vi "Teleop Fingers.vi"(10 "Joystick Data":T2, 11 "Arm Out":T1) -> ()   [LabVIEW 2013]
uses:
  Joystick Data.ctl
  <vilib>/Rock Robotics/WPI/Solenoid/WPI_SolenoidValue.ctl
  <vilib>/Rock Robotics/WPI/Solenoid/WPI_SolenoidSetEnum.vi
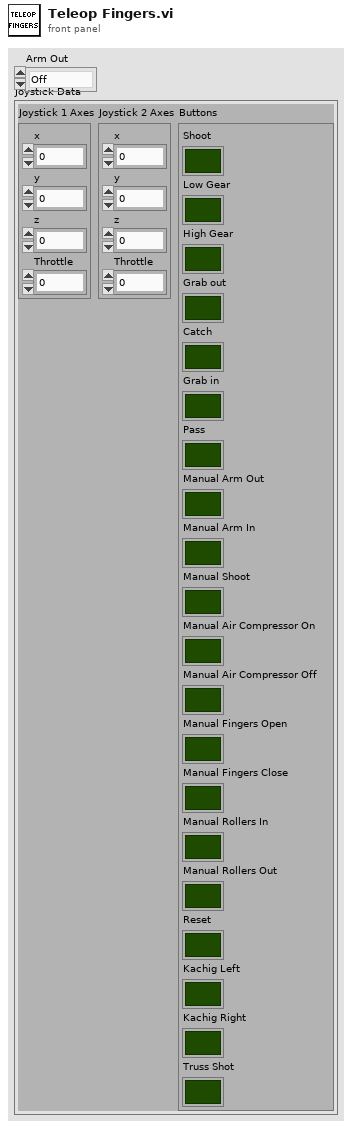
[diagram p1: front panel]
types:
  T1 = typedef "WPI_SolenoidValue.ctl" = enum16{"Off", "On", "Forward", "Reverse"}
  T2 = typedef "Joystick Data.ctl" = cluster{"Joystick 1 Axes":cluster{"x":dbl, "y":dbl, "z":dbl, "Throttle":dbl}, "Joystick 2 Axes":cluster{"x":dbl, "y":dbl, "z":dbl, "Throttle":dbl}, "Buttons":cluster{"Shoot":bool, "Low Gear":bool, "High Gear":bool, "Grab out":bool, "Catch":bool, "Grab in":bool, "Pass":bool, "Manual Arm Out":bool, "Manual Arm In":bool, "Manual Shoot":bool, "Manual Air Compressor On":bool, "Manual Air Compressor Off":bool, "Manual Fingers Open":bool, "Manual Fingers Close":bool, "Manual Rollers In":bool, "Manual Rollers Out":bool, "Reset":bool, "Kachig Left":bool, "Kachig Right":bool, "Truss Shot":bool}}
  T3 = typedef "WPI_SolenoidDevRef.ctl" = cluster{"DevStatus":errorcluster, "Solenoid Module":T4, "Forward Solenoid Channel":T5, "Reverse Solenoid Channel":T5}
  T4 = typedef "FPGA_TypedefSolenoidModule.ctl" = enum16{"Solenoid Module 1", "Solenoid Module 2"}
  T5 = typedef "WPI_SolenoidChannel.ctl" = enum8{"Solenoid 1", "Solenoid 2", "Solenoid 3", "Solenoid 4", "Solenoid 5", "Solenoid 6", "Solenoid 7", "Solenoid 8", "Invalid"}
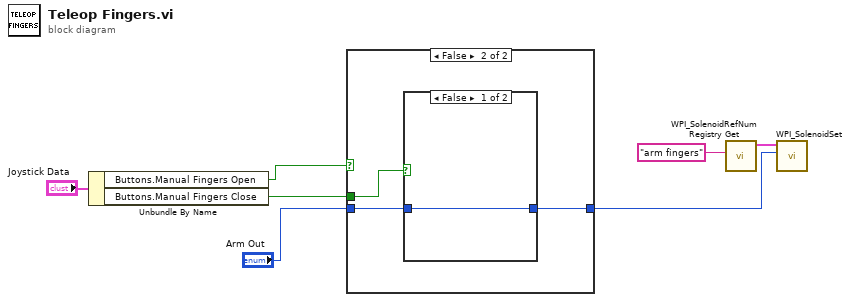
[diagram p0: block diagram]
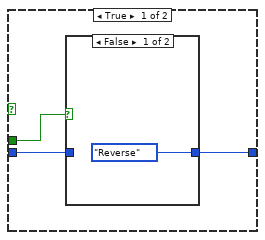
[diagram p2: hidden frame]
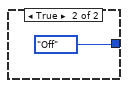
[diagram p3: hidden frame]
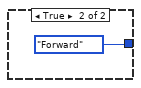
[diagram p4: hidden frame]
diagram:
  n1 = Unbundle By Name("Joystick Data") -> ("Buttons.Manual Fingers Open"=w4:bool, "Buttons.Manual Fingers Close"=w3:bool)
  n2 = case shown="False" w4 {
    tunnel: w3 -> [w10 w15]
    tunnel: "Arm Out" -> [w9 w14]
    tunnel: [w8 w13] -> w1
    frame True {
      n3 = case shown="False" w10 {
        tunnel: [WPI_SolenoidValue."Reverse" ("Arm Out") WPI_SolenoidValue."Off" ("Arm Out")] -> w8
        tunnel: w9 -> [_ _]
        frame False {
        }
        frame True {
        }
      }
    }
    frame False {
      n4 = case shown="False" w15 {
        tunnel: w14 -> [w16 _]
        tunnel: [w16 WPI_SolenoidValue."Forward" ("Arm Out")] -> w13
        frame False {
        }
        frame True {
        }
      }
    }
  }
  n5 = call <vilib>:"WPI_SolenoidRefNum Registry Get.vi"("refnum name"="arm fingers") -> ("SolenoidDevRef"=w7:T3)  [unwired: 9 in, 1 out]
  n6 = call-poly <vilib>:"WPI_SolenoidSet.vi"("Value"=w1, "SolenoidDevRef"=w7) -> ()  [unwired: 8 in, 2 out]
